vi "startCycle.vi"(8 "error in (no error)":errorcluster, 11 "OvenController in":refnum<class "OvenController.lvclass">) -> (0 "error out":errorcluster, 3 "OvenController out":refnum<class "OvenController.lvclass">)   [LabVIEW 2023, in "AbstractFactory.lvlib" / "OvenController.lvclass"]
uses:
  OvenController.lvclass
  OvenController.lvclass/OvenController.ctl
  IConnection/IConnection.lvclass
  ICommandBuilder/ICommandBuilder.lvclass
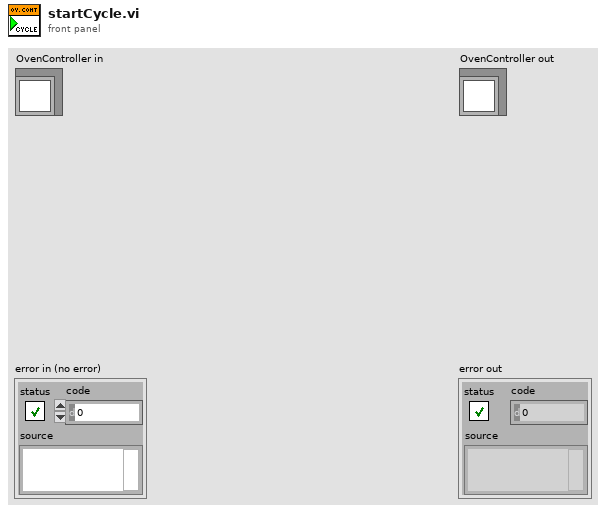
[diagram p1: front panel]
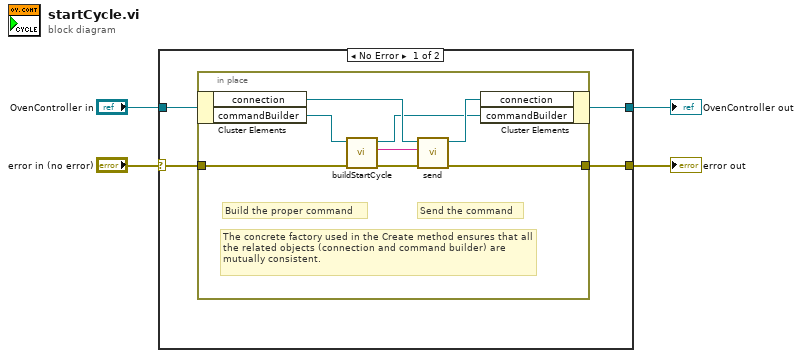
[diagram p0: block diagram]
diagram:
  n1 = case shown="No Error" "error in (no error)" {
    selector: "error in (no error)" -> [w6 w18]
    tunnel: [w5 w18] -> w3
    tunnel: [w8 w17] -> w1
    tunnel: "OvenController in" -> [w7 w17]
    frame No Error {
      n2 = in-place {
        in-place-border: w6 -> [w11]
        in-place-border: [w14] -> w5
        # "The concrete factory used in the Create method ensures that all the related objects (connection and command builder) are mutually consistent."
        # "Send the command"
        # "Build the proper command"
        n3 = in-place-cluster #1(w7) -> ("connection"=w16:refnum<class "IConnection.lvclass">, "commandBuilder"=w13:refnum<class "ICommandBuilder.lvclass">)
        n4 = call-dynamic "buildStartCycle.vi"("error in (no error)"=w11, "ICommandBuilder in"=w13) -> ("error out"=w12:errorcluster, "message"=w9:string, "ICommandBuilder out"=w10:refnum<class "ICommandBuilder.lvclass">)  [unwired: 7 in]
        n5 = call-dynamic "send.vi"("error in (no error)"=w12, "message"=w9, "IConnection in"=w16) -> ("error out"=w14:errorcluster, "IConnection out"=w15:refnum<class "IConnection.lvclass">)  [unwired: 7 in]
        n6 = in-place-cluster #1("connection"=w15, "commandBuilder"=w10) -> (w8:refnum<class "OvenController.lvclass">)
      }
    }
    frame Error {
    }
  }
  "error out" <- w3
  "OvenController out" <- w1
